vi "ROS_Topic_Write_Primitive.vi"(2 "Msg in":string, 3 "ROS in":T1={"topic port"=0, "Node"="", "topic"="", "type"="", "node port"=0, "error "={"status"=FALSE, "code"=0, "source"=""}, "Direction"=enum."Node", "APIs"=[], "Update (ms)"=1, "write queue"=1}) -> (1 "ROS out":T1={"topic port"=0, "Node"="", "topic"="", "type"="", "node port"=0, "error "={"status"=FALSE, "code"=0, "source"=""}, "Direction"=enum."Node", "APIs"=[], "Update (ms)"=1, "write queue"=1})   [LabVIEW 2012]
doc: "Writes the data to background server when publishing data or sending service calls. Implemented in ROS_Topic_Write and ROS_Topic_Write_Continuous."
uses:
  <userlib>/ROSforLV/ROS/Code/SubVIs/_ROSControl.ctl
  <userlib>/ROSforLV/ROS/Code/SubVIs/_ROSDirection.ctl
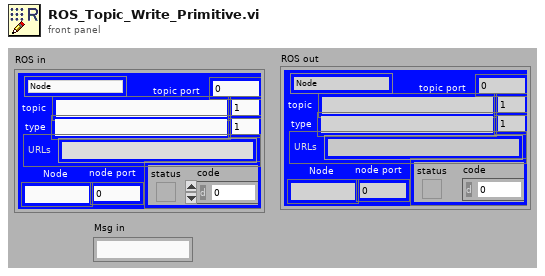
[diagram p1: front panel]
types:
  T1 = typedef "_ROSControl.ctl" = cluster{"topic port":u16, "Node":string, "topic":string, "type":string, "node port":u16, "error ":errorcluster, "Direction":T2, "APIs":string[], "Update (ms)":u16, "write queue":u16}
  T2 = typedef "_ROSDirection.ctl" = enum16{"Node", "Publisher", "Subscriber", "Service Client"}
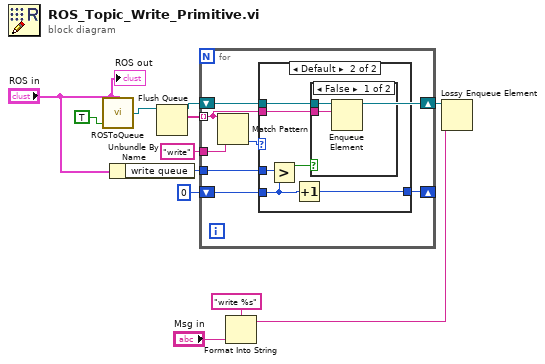
[diagram p0: block diagram]
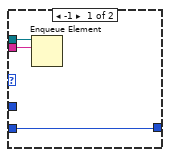
[diagram p2: hidden frame]
diagram:
  n1 = call <userlib>:"ROSToQueue.vi"("Wait?"=TRUE, "ROS"="ROS in") -> ("queue"=w6:refnum<queue>)  [unwired: 2 in, 1 out]
  n2 = Unbundle By Name("ROS in") -> ("write queue"=w2:u16)
  n3 = Flush Queue(queue=w6) -> (queue out=w8:refnum<queue>, remaining elements=w10:string[])  [unwired: 1 in, 1 out]
  n4 = for {
    tunnel: w10 -> [w17] mode=indexing
    tunnel: "write" ("regular expression") -> [w19]
    shift-right: [w13] -> _
    shift-left: u32 0 -> [w14]
    tunnel: w2 -> [w15]
    shift-right: [w16] -> w5
    shift-left: w8 -> [w16]
    n5 = Match Pattern(string=w17, regular expression=w19) -> (offset past match=w18:i32)  [unwired: 1 in, 3 out]
    n6 = case shown="Default" w18 {
      tunnel: w17 -> [w22 w23]
      tunnel: w16 -> [w21 w24]
      tunnel: w15 -> [_ w28]
      tunnel: w14 -> [w20 w27]
      tunnel: [w20 w26] -> w13
      frame -1 {
        n7 = Enqueue Element(queue=w21, element=w22) -> ()  [unwired: 2 in, 3 out]
      }
      frame Default {
        n8 = Greater?(x=w28, y=w27) -> (0:w25:bool)
        n9 = Increment(x=w27) -> (x+1=w26:u32)
        n10 = case shown="False" w25 {
          tunnel: w24 -> [w30 _]
          tunnel: w23 -> [w29 _]
          frame False {
            n11 = Enqueue Element(queue=w30, element=w29) -> ()  [unwired: 2 in, 3 out]
          }
          frame True {
          }
        }
      }
    }
  }
  n12 = Format Into String(format string="write %s" ("name (unnamed)"), "Msg in") -> (resulting string=w4:string)  [unwired: 2 in, 1 out]
  n13 = Lossy Enqueue Element(queue=w5, element=w4) -> ()  [unwired: 1 in, 4 out]
  "ROS out" <- "ROS in"
